vi "Save.vi"(8 "error in (no error)":errorcluster, 9 "Automatic?":bool, 10 "configuration file path":path, 11 "SettingsFile in":refnum<class "SettingsFile.lvclass">) -> (0 "error out":errorcluster, 3 "SettingsFile out":refnum<class "SettingsFile.lvclass">)   [LabVIEW 2018, in "SettingsFile.lvclass"]
uses:
  SettingsFile.lvclass
  SettingsFile.lvclass/SettingsFile.ctl
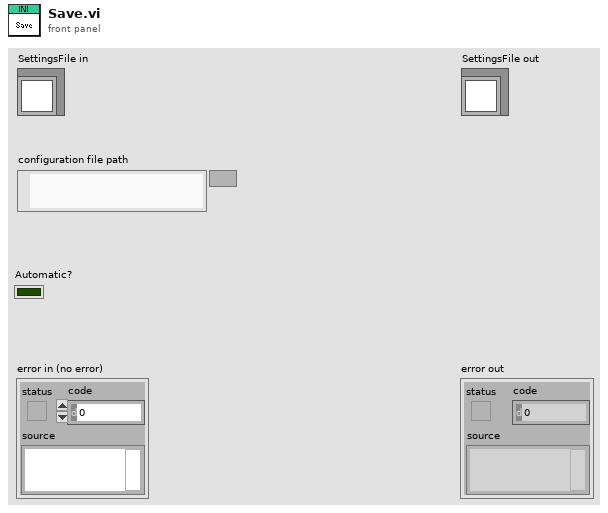
[diagram p1: front panel]
types:
  T1 = typedef "Graph_references.ctl" = cluster{"upper":T2, "lower":T2, "Freq graph":refnum<vi>, "Adaptive FF graph":refnum<vi>}
  T2 = typedef "graph_controls.ctl" = cluster{"Graph":refnum<vi>, "Time btn":refnum<vi>, "Amplitude btn":refnum<vi>, "Chart":refnum<vi>}
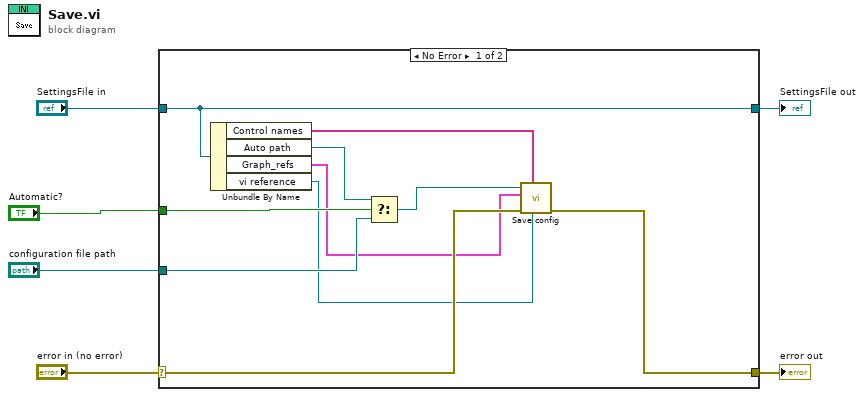
[diagram p0: block diagram]
diagram:
  n1 = case shown="No Error" "error in (no error)" {
    selector: "error in (no error)" -> [w10 w18]
    tunnel: [w9 w18] -> w5
    tunnel: [w16 w17] -> w3
    tunnel: "SettingsFile in" -> [w16 w17]
    tunnel: "Automatic?" -> [w14 _]
    tunnel: "configuration file path" -> [w12 _]
    frame No Error {
      n2 = Unbundle By Name(w16) -> ("Control names"=w15:string[], "Auto path"=w13:path, "Graph_refs"=w8:T1, "vi reference"=w7:refnum<vi>)
      n3 = Select(t=w13, s=w14, f=w12) -> (s? t:f=w11:path)
      n4 = call "Save config.vi"("VI ref"=w7, "Control names"=w15, "error in (no error)"=w10, "Graph_refs"=w8, "configuration file path"=w11) -> ("error out"=w9:errorcluster)  [unwired: 6 in]
    }
    frame Error {
    }
  }
  "error out" <- w5
  "SettingsFile out" <- w3
